vi "DemoDataLineGraphs.vi"() -> (1 "XY Graph 3":cluster{"X":dbl[], "Y":dbl[]}[](array[cluster]), 2 "XY Graph 2":cluster{"X":dbl[], "Y":dbl[]}[](array[cluster]), 3 "XY Graph 3":cluster{"X":dbl[], "Y":dbl[]}[](array[cluster]))   [LabVIEW 2022 SP3]
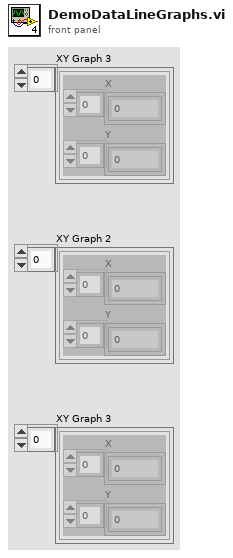
[diagram p1: front panel]
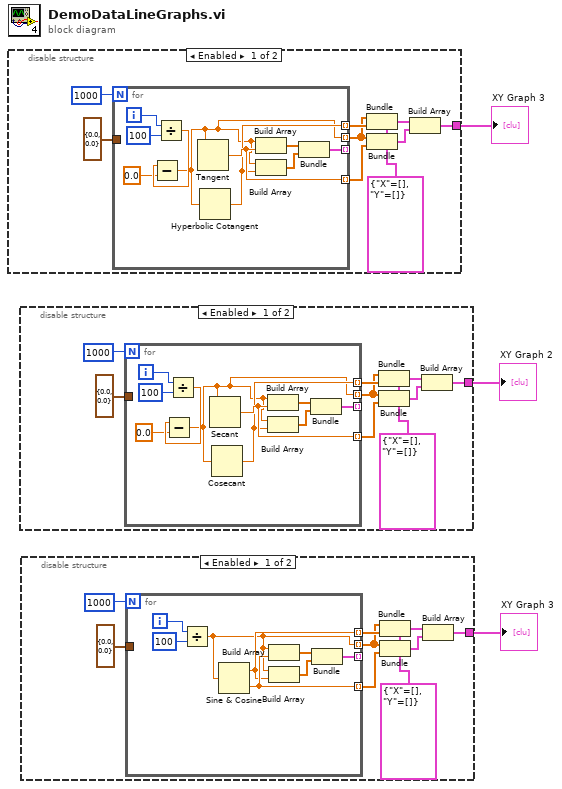
[diagram p0: block diagram]
diagram:
  n1 = disable-structure shown="Enabled" {
    disable-tunnel: [w4 _] -> w2
    frame Enabled {
      w5 = cluster{"X":dbl[], "Y":dbl[]} {"X"=[], "Y"=[]} ("output cluster")
      n2 = for {
        N: 1000 -> [_]
        tunnel: [w16] -> w9 mode=indexing
        tunnel: [w17] -> w10 mode=indexing
        tunnel: [w13] -> w8 mode=indexing
        tunnel: cluster{"X":dbl, "Y":dbl} {"X"=0.0, "Y"=0.0} -> [_]
        tunnel: [w18] -> _ mode=indexing
        i -> [w22]
        n3 = Divide(x=w22, y=100) -> (x/y=w15:dbl)
        n4 = Subtract(x=w15, y=0.0) -> (x-y=w13:dbl)
        n5 = Tangent(1:w13) -> (0:w17:dbl)
        n6 = Hyperbolic Cotangent(1:w13) -> (0:w16:dbl)
        n7 = Build Array(w13, w17) -> (w20:dbl[])
        n8 = Build Array(w13, w16) -> (w19:dbl[])
        n9 = Bundle(w20, w19) -> (w18:cluster{dbl[], dbl[]})  [unwired: 1 in]
      }
      n10 = Bundle(cluster=w5, "X"=w8, "Y"=w9) -> (w6:cluster{"X":dbl[], "Y":dbl[]})
      n11 = Bundle(cluster=w5, "X"=w8, "Y"=w10) -> (w7:cluster{"X":dbl[], "Y":dbl[]})
      n12 = Build Array(w6, w7) -> (w4:cluster{"X":dbl[], "Y":dbl[]}[])
    }
    frame Disabled {
    }
  }
  "XY Graph 3" <- w2
  n13 = disable-structure shown="Enabled" {
    disable-tunnel: [w23 _] -> w1
    frame Enabled {
      w24 = cluster{"X":dbl[], "Y":dbl[]} {"X"=[], "Y"=[]} ("output cluster")
      n14 = for {
        N: 1000 -> [_]
        tunnel: [w35] -> w28 mode=indexing
        tunnel: [w36] -> w29 mode=indexing
        tunnel: [w32] -> w27 mode=indexing
        tunnel: cluster{"X":dbl, "Y":dbl} {"X"=0.0, "Y"=0.0} -> [_]
        tunnel: [w37] -> _ mode=indexing
        i -> [w41]
        n15 = Divide(x=w41, y=100) -> (x/y=w34:dbl)
        n16 = Subtract(x=w34, y=0.0) -> (x-y=w32:dbl)
        n17 = Secant(1:w32) -> (0:w36:dbl)
        n18 = Cosecant(1:w32) -> (0:w35:dbl)
        n19 = Build Array(w32, w36) -> (w39:dbl[])
        n20 = Build Array(w32, w35) -> (w38:dbl[])
        n21 = Bundle(w39, w38) -> (w37:cluster{dbl[], dbl[]})  [unwired: 1 in]
      }
      n22 = Bundle(cluster=w24, "X"=w27, "Y"=w28) -> (w25:cluster{"X":dbl[], "Y":dbl[]})
      n23 = Bundle(cluster=w24, "X"=w27, "Y"=w29) -> (w26:cluster{"X":dbl[], "Y":dbl[]})
      n24 = Build Array(w25, w26) -> (w23:cluster{"X":dbl[], "Y":dbl[]}[])
    }
    frame Disabled {
    }
  }
  "XY Graph 2" <- w1
  n25 = disable-structure shown="Enabled" {
    disable-tunnel: [w42 _] -> w3
    frame Enabled {
      w43 = cluster{"X":dbl[], "Y":dbl[]} {"X"=[], "Y"=[]} ("output cluster")
      n26 = for {
        N: 1000 -> [_]
        tunnel: [w55] -> w47 mode=indexing
        tunnel: [w56] -> w48 mode=indexing
        tunnel: [w51] -> w46 mode=indexing
        tunnel: cluster{"X":dbl, "Y":dbl} {"X"=0.0, "Y"=0.0} -> [_]
        tunnel: [w52] -> _ mode=indexing
        i -> [w58]
        n27 = Divide(x=w58, y=100) -> (x/y=w51:dbl)
        n28 = Sine & Cosine(0:w51) -> (1:w55:dbl, 2:w56:dbl)
        n29 = Build Array(w51, w56) -> (w54:dbl[])
        n30 = Build Array(w51, w55) -> (w53:dbl[])
        n31 = Bundle(w54, w53) -> (w52:cluster{dbl[], dbl[]})  [unwired: 1 in]
      }
      n32 = Bundle(cluster=w43, "X"=w46, "Y"=w47) -> (w44:cluster{"X":dbl[], "Y":dbl[]})
      n33 = Bundle(cluster=w43, "X"=w46, "Y"=w48) -> (w45:cluster{"X":dbl[], "Y":dbl[]})
      n34 = Build Array(w44, w45) -> (w42:cluster{"X":dbl[], "Y":dbl[]}[])
    }
    frame Disabled {
    }
  }
  "XY Graph 3" <- w3
